vi "CC Parse Right Ascension.vi"(8 "error in (no error)":errorcluster, 11 "Right Ascension string":string) -> (0 "error out":errorcluster, 2 "Angle":dbl, 3 "Right Ascension cluster":T1)   [LabVIEW 2021]
uses:
  <vilib>/regexp/Match Regular Expression.xnode
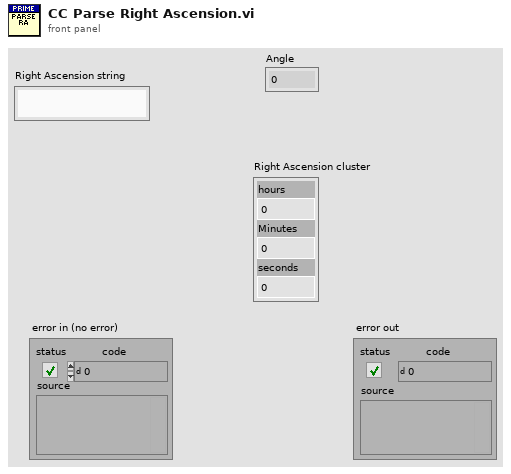
[diagram p1: front panel]
types:
  T1 = cluster{"hours":dbl, "Minutes":dbl, "seconds":dbl}
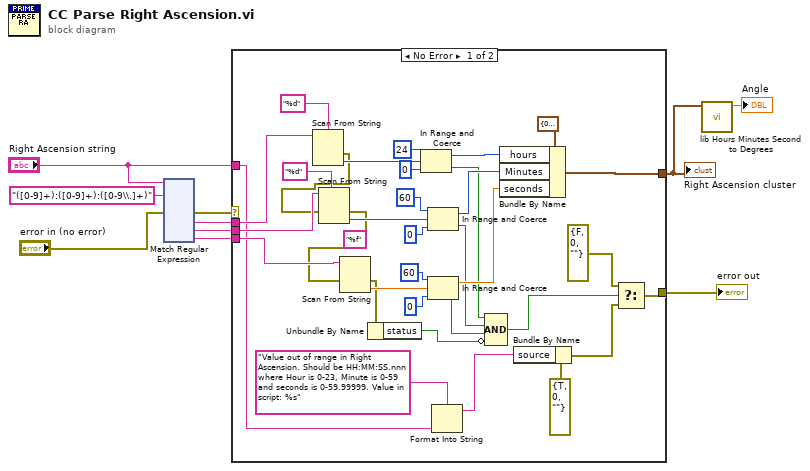
[diagram p0: block diagram]
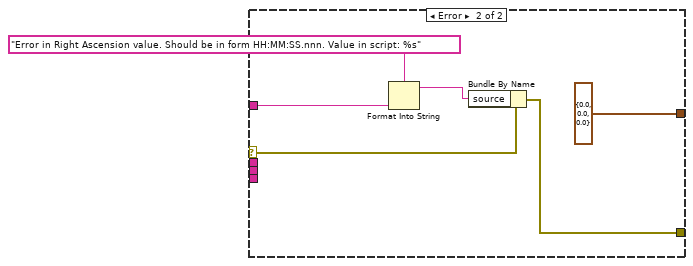
[diagram p2: hidden frame]
diagram:
  n1 = xnode "Match Regular Expression"("input string"="Right Ascension string", "regular expression"="([0-9]+):([0-9]+):([0-9\\.]+)", "error in"="error in (no error)") -> ("error out"=w5:errorcluster, "submatch 1"=w9:string, "submatch 2"=w8:string, "submatch 3"=w7:string)  [unwired: 3 in, 4 out]
  n2 = case shown="No Error" w5 {
    selector: w5 -> [_ w48]
    tunnel: w9 -> [w44 _]
    tunnel: w8 -> [w41 _]
    tunnel: w7 -> [w40 _]
    tunnel: [w26 T1 {"hours"=0.0, "Minutes"=0.0, "seconds"=0.0} ("Right Ascension 2")] -> w2
    tunnel: "Right Ascension string" -> [w18 w49]
    tunnel: [w16 w46] -> w3
    frame No Error {
      (unwired) "%f" ("format string")
      n3 = Scan From String(format string="%d", input string=w44) -> (error out=w15:errorcluster, output 1=w39:i32)  [unwired: 3 in, 2 out]
      n4 = Scan From String(format string="%d", input string=w41, error in=w15) -> (error out=w14:errorcluster, output 1=w36:i32)  [unwired: 2 in, 2 out]
      n5 = Scan From String(input string=w40, error in=w14) -> (error out=w13:errorcluster, output 1=w31:dbl)  [unwired: 3 in, 2 out]
      n6 = Unbundle By Name(w13) -> ("status"=w12:bool)
      n7 = In Range and Coerce(upper limit=24, x=w39, lower limit=0) -> (coerced(x)=w29:i32, In Range?=w25:bool)
      n8 = In Range and Coerce(upper limit=60, x=w36, lower limit=0) -> (coerced(x)=w28:i32, In Range?=w24:bool)
      n9 = In Range and Coerce(upper limit=60, x=w31, lower limit=0) -> (coerced(x)=w27:dbl, In Range?=w23:bool)
      n10 = Format Into String(format string="Value out of range in Right Ascension. Should be HH:MM:SS.nnn where Hour is 0-23, Minute is 0-59 and seconds is 0-59.99999. Value in script: %s", w18) -> (resulting string=w17:string)  [unwired: 2 in, 1 out]
      n11 = Compound Arithmetic op=AND(w25, w24, w23, invert w12) -> (w22:bool)
      n12 = Bundle By Name(cluster=T1 {"hours"=0.0, "Minutes"=0.0, "seconds"=0.0} ("Right Ascension 2"), "hours"=w29, "Minutes"=w28, "seconds"=w27) -> (w26:T1)
      n13 = Bundle By Name(cluster=errorcluster {"status"=TRUE, "code"=0, "source"=""} ("error out"), "source"=w17) -> (w20:errorcluster)
      n14 = Select(t=errorcluster {"status"=FALSE, "code"=0, "source"=""} ("error out"), s=w22, f=w20) -> (s? t:f=w16:errorcluster)
    }
    frame Error {
      n15 = Format Into String(format string="Error in Right Ascension value. Should be in form HH:MM:SS.nnn. Value in script: %s", w49) -> (resulting string=w47:string)  [unwired: 2 in, 1 out]
      n16 = Bundle By Name(cluster=w48, "source"=w47) -> (w46:errorcluster)
    }
  }
  "error out" <- w3
  "Right Ascension cluster" <- w2
  n17 = call "lib Hours Minutes Second to Degrees.vi"("Right Ascension cluster"=w2) -> ("Angle"=→"Angle":dbl)  [unwired: 9 in, 1 out]
